vi "NucleationField.vi"(3 "array":dbl[](array[numeric])) -> (0 "Nucleation Field Downwards":dbl, 1 "Nucleation Field Upwards":dbl)   [LabVIEW 2019]
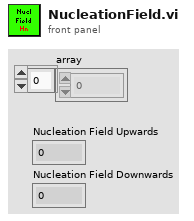
[diagram p1: front panel]
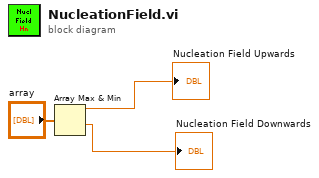
[diagram p0: block diagram]
diagram:
  n1 = Array Max & Min(array="array") -> (max value=→"Nucleation Field Upwards":dbl, min value=→"Nucleation Field Downwards":dbl)  [unwired: 2 out]
